vi "Teleop.vi"(10 "Match Info":T1={"Autonomous Elapsed Seconds"=0.0, "TeleOp Elapsed Seconds"=0.0, "Disabled Elapsed Seconds"=0.0, "Visited Autonomous"=FALSE, "Visited TeleOp"=FALSE, "Visited Disabled"=FALSE, "Autonomous Settings"={"Autonomous Style"=enum."Independent", "VI Refnum"=refnum}}, 11 "Call Context":T2) -> ()   [LabVIEW 2019]
doc: "This VI is called for each enabled TeleOp packet received from the DS. It is typically used to read from joysticks and other inputs and update I/O or setpoints for timed control loops. It should complete and return within 20 milliseconds or risk missing DS packets."
uses:
  <vilib>/Rock Robotics/WPI/DriverStation/WPI_DriverStationDerivedRobotMode.ctl
  <vilib>/Rock Robotics/WPI/DriverStation/WPI_DriverStationMatch Info.ctl
  Framework/Robot Global Data.vi
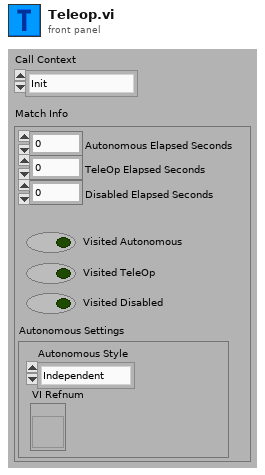
[diagram p1: front panel]
types:
  T1 = typedef "WPI_DriverStationMatch Info.ctl" = cluster{"Autonomous Elapsed Seconds":dbl, "TeleOp Elapsed Seconds":dbl, "Disabled Elapsed Seconds":dbl, "Visited Autonomous":bool, "Visited TeleOp":bool, "Visited Disabled":bool, "Autonomous Settings":cluster{"Autonomous Style":enum16{"Iterative", "Independent"}, "VI Refnum":refnum<vi>}}
  T2 = typedef "WPI_DriverStationDerivedRobotMode.ctl" = enum16{"Init", "Execute", "Stop"}
  T3 = typedef "Command Status Info.ctl" = cluster{"Name":string, "Status":T4, "notifier out":T5}
  T4 = typedef "Completion Status.ctl" = enum16{"Successful", "Aborted", "Incomplete"}
  T5 = typedef "Completion Notifier.ctl" = refnum<notifier>
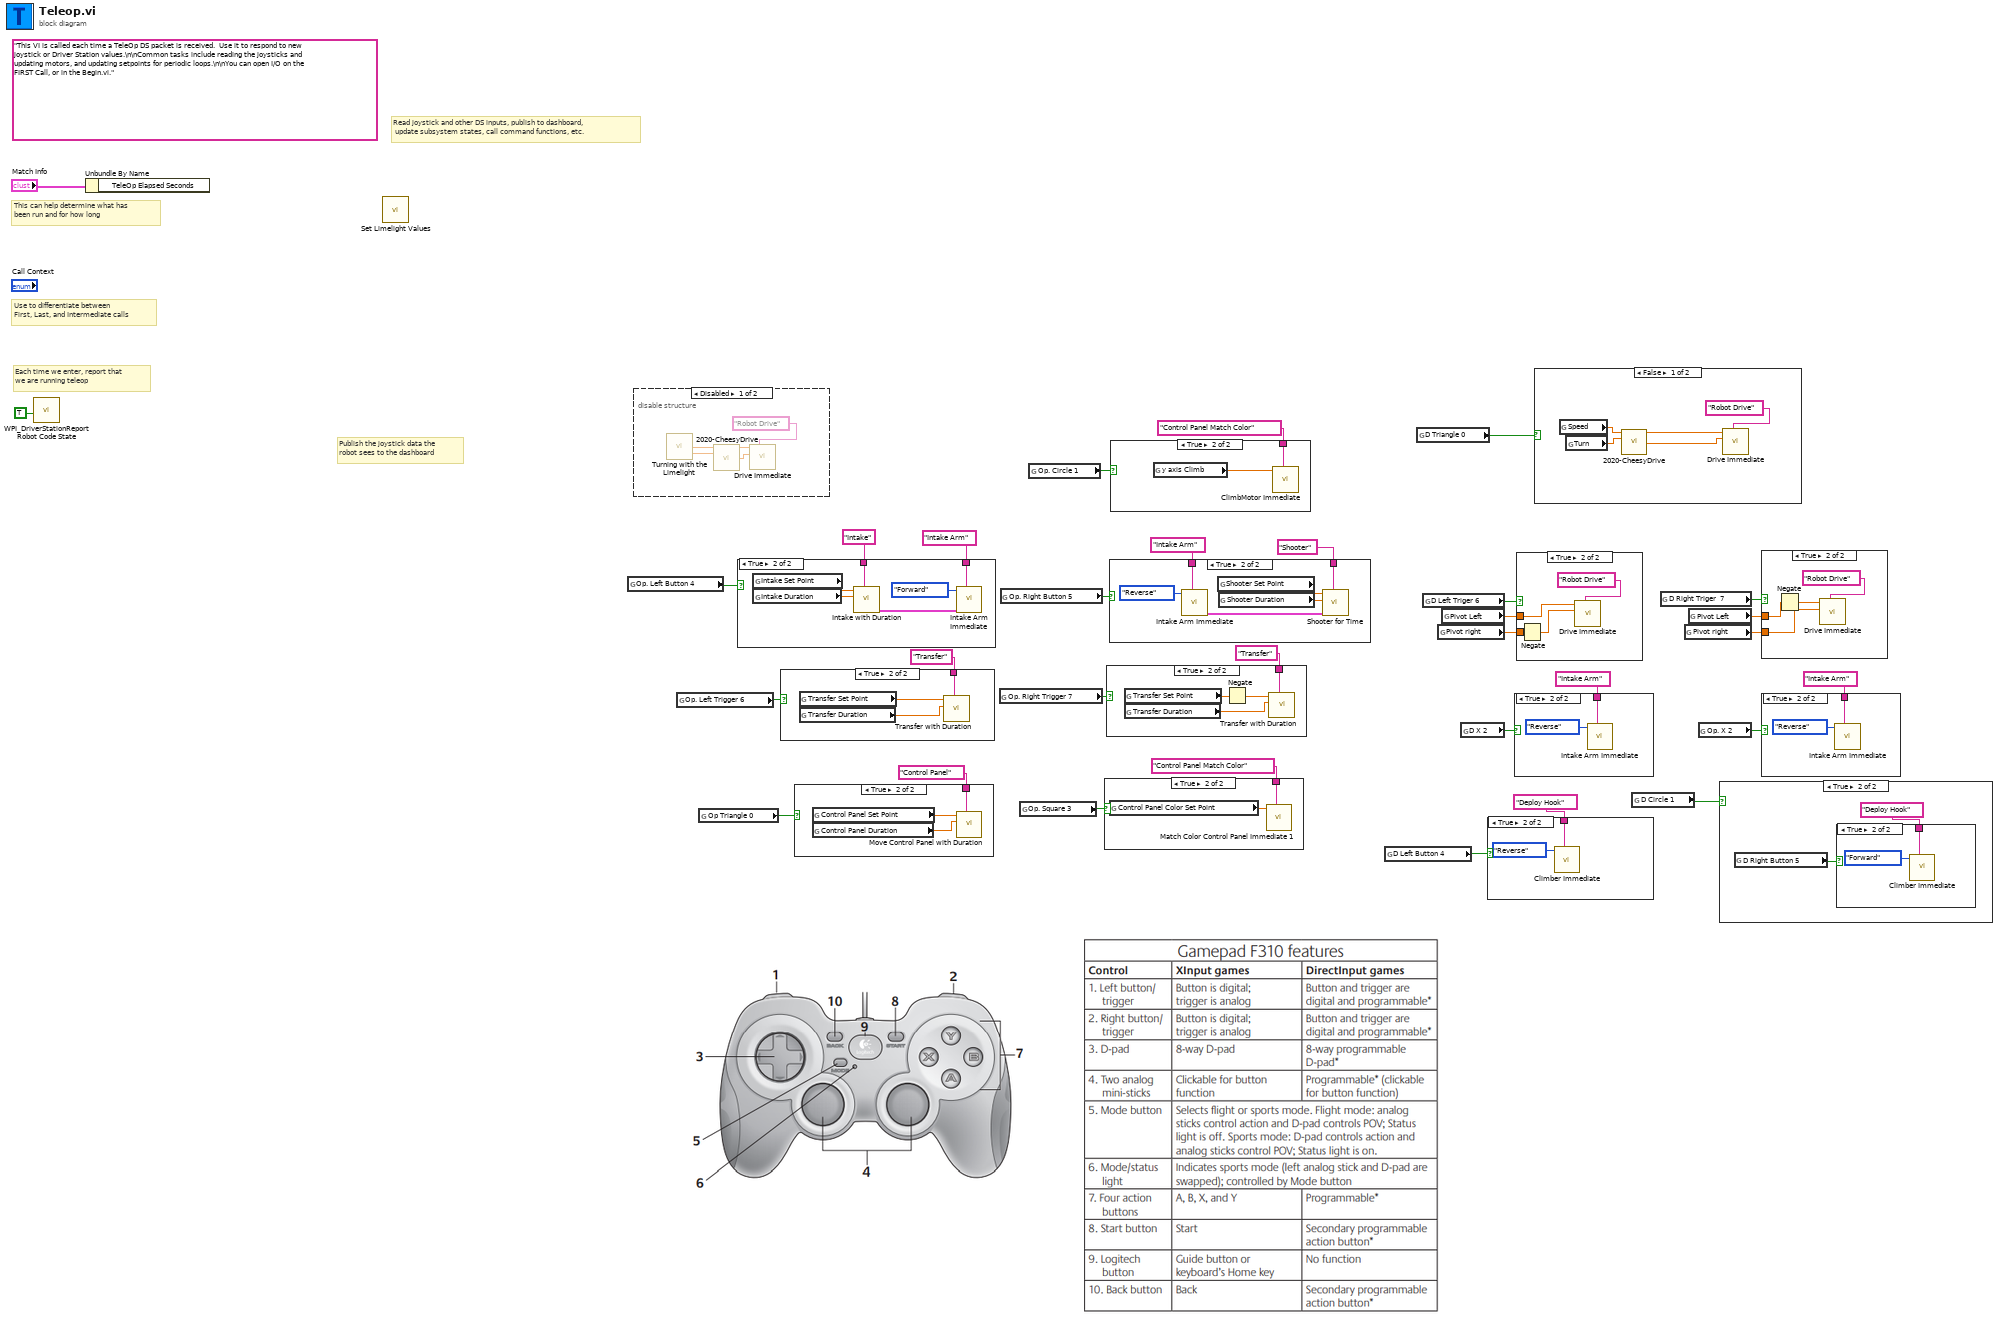
[diagram p0: block diagram]
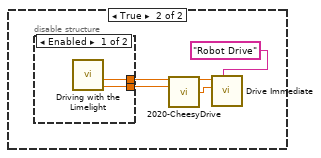
[diagram p8: hidden frame]
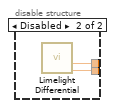
[diagram p9: hidden frame]
diagram:
  (unwired) "This VI is called each time a TeleOp DS packet is received.  Use it to respond to new joystick or Driver Station values.\n\nCommon tasks include reading the joysticks and updating motors, and updating setpoints for periodic loops.\n\nYou can open I/O on the FIRST Call, or in the Begin.vi."
  # "Publish the joystick data the\nrobot sees to the dashboard"
  # "Read joystick and other DS inputs, publish to dashboard,\n update subsystem states, call command functions, etc."
  # "Each time we enter, report that\nwe are running teleop"
  # "Use to differentiate between\nFirst, Last, and Intermediate calls"
  # "This can help determine what has\nbeen run and for how long"
  n1 = call <vilib>:"WPI_DriverStationReport Robot Code State.vi"("TeleOp"=TRUE ("Autonomous")) -> ()  [unwired: 10 in, 1 out]
  n2 = Unbundle By Name("Match Info") -> ()  [unwired: 1 out]
  n3 = call "Set Limelight Values.vi"() -> ()  [unwired: 12 in]
  n4 = global read "Robot Global Data.vi" "Op. Left Button 4"() -> (w30:bool)
  n5 = disable-structure shown="Disabled" {
    frame Disabled {
      n6 = call "Turning with the Limelight.vi"() -> ("TurnCommand"=w36:dbl, "Speed Command"=w37:dbl)  [unwired: 9 in, 1 out]
      n7 = call "2020-CheesyDrive.vi"("Throttle"=w37, "Wheel"=w36) -> ("Left PWM"=w35:dbl, "Right PWM"=w34:dbl)  [unwired: 12 in]
      n8 = call "Drive Immediate.vi"("Description"="Robot Drive", "Right Setpoint"=w34, "Left Setpoint"=w35) -> ()  [unwired: 8 in, 1 out]
    }
    frame Enabled {
    }
  }
  n9 = global read "Robot Global Data.vi" "Op. Left Trigger 6"() -> (w24:bool)
  n10 = global read "Robot Global Data.vi" "Op Triangle 0"() -> (w17:bool)
  n11 = case shown="True" w30 {
    tunnel: "Intake" ("refnum name") -> [_ w43]
    tunnel: "Intake Arm" ("refnum name") -> [_ w39]
    frame False {
    }
    frame True {
      n12 = global read "Robot Global Data.vi" "Intake Set Point"() -> (w42:dbl)
      n13 = global read "Robot Global Data.vi" "Intake Duration"() -> (w41:dbl)
      n14 = call "Intake with Duration.vi"("Description"=w43, "Duration (s)"=w41, "Setpoint"=w42) -> ("Command Info Out"=w38:T3)  [unwired: 8 in]
      n15 = call "Intake Arm Immediate.vi"("Description"=w39, "Command Info In"=w38, "Relay Value"=enum16{"Off", "On", "Forward", "Reverse"}."Forward") -> ()  [unwired: 8 in, 1 out]
    }
  }
  n16 = case shown="True" w24 {
    tunnel: "Transfer" ("refnum name") -> [_ w46]
    frame False {
    }
    frame True {
      n17 = global read "Robot Global Data.vi" "Transfer Set Point"() -> (w45:dbl)
      n18 = global read "Robot Global Data.vi" "Transfer Duration"() -> (w44:dbl)
      n19 = call "Transfer with Duration.vi"("Description"=w46, "Duration (s)"=w44, "Setpoint"=w45) -> ()  [unwired: 8 in, 1 out]
    }
  }
  n20 = case shown="True" w17 {
    tunnel: "Control Panel" ("refnum name") -> [_ w49]
    frame False {
    }
    frame True {
      n21 = global read "Robot Global Data.vi" "Control Panel Set Point"() -> (w48:dbl)
      n22 = global read "Robot Global Data.vi" "Control Panel Duration"() -> (w47:dbl)
      n23 = call "Move Control Panel with Duration.vi"("Description"=w49, "Duration (s)"=w47, "Setpoint"=w48) -> ()  [unwired: 8 in, 1 out]
    }
  }
  n24 = global read "Robot Global Data.vi" "Op. Right Trigger 7"() -> (w25:bool)
  n25 = global read "Robot Global Data.vi" "Op. Right Button 5"() -> (w26:bool)
  n26 = global read "Robot Global Data.vi" "Op. Square 3"() -> (w14:bool)
  n27 = global read "Robot Global Data.vi" "Op. Circle 1"() -> (w2:bool)
  n28 = case shown="True" w14 {
    tunnel: "Control Panel Match Color" ("refnum name") -> [_ w51]
    frame False {
    }
    frame True {
      n29 = global read "Robot Global Data.vi" "Control Panel Color Set Point"() -> (w50:dbl)
      n30 = call "Match Color Control Panel Immediate 1.vi"("Description"=w51, "Setpoint"=w50) -> ()  [unwired: 9 in, 1 out]
    }
  }
  n31 = case shown="True" w25 {
    tunnel: "Transfer" ("refnum name") -> [_ w55]
    frame False {
    }
    frame True {
      n32 = global read "Robot Global Data.vi" "Transfer Set Point"() -> (w53:dbl)
      n33 = global read "Robot Global Data.vi" "Transfer Duration"() -> (w52:dbl)
      n34 = Negate(x=w53) -> (-x=w54:dbl)
      n35 = call "Transfer with Duration.vi"("Description"=w55, "Duration (s)"=w52, "Setpoint"=w54) -> ()  [unwired: 8 in, 1 out]
    }
  }
  n36 = case shown="True" w26 {
    tunnel: "Shooter" ("refnum name") -> [_ w61]
    tunnel: "Intake Arm" ("refnum name") -> [_ w56]
    frame False {
    }
    frame True {
      n37 = call "Intake Arm Immediate.vi"("Description"=w56, "Relay Value"=enum16{"Off", "On", "Forward", "Reverse"}."Reverse") -> ("Command Info Out"=w57:T3)  [unwired: 9 in]
      n38 = global read "Robot Global Data.vi" "Shooter Set Point"() -> (w60:dbl)
      n39 = global read "Robot Global Data.vi" "Shooter Duration"() -> (w59:dbl)
      n40 = call "Shooter for Time.vi"("Description"=w61, "Command Info In"=w57, "Duration (s)"=w59, "Setpoint"=w60) -> ()  [unwired: 7 in, 1 out]
    }
  }
  n41 = case shown="True" w2 {
    tunnel: "Control Panel Match Color" ("refnum name") -> [_ w63]
    frame False {
    }
    frame True {
      n42 = global read "Robot Global Data.vi" "y axis Climb"() -> (w62:dbl)
      n43 = call "ClimbMotor Immediate.vi"("Description"=w63, "Setpoint"=w62) -> ()  [unwired: 9 in, 1 out]
    }
  }
  n44 = global read "Robot Global Data.vi" "D Left Button 4"() -> (w7:bool)
  n45 = global read "Robot Global Data.vi" "D Triangle 0"() -> (w8:bool)
  n46 = global read "Robot Global Data.vi" "D Left Triger 6"() -> (w22:bool)
  n47 = global read "Robot Global Data.vi" "Pivot right"() -> (w11:dbl)
  n48 = global read "Robot Global Data.vi" "Pivot Left"() -> (w12:dbl)
  n49 = global read "Robot Global Data.vi" "D X 2"() -> (w15:bool)
  n50 = case shown="True" w7 {
    tunnel: "Deploy Hook" ("refnum name") -> [_ w64]
    frame False {
    }
    frame True {
      n51 = call "Climber Immediate.vi"("Description"=w64, "Value"=enum16{"Off", "On", "Forward", "Reverse"}."Reverse" ("Relay Value")) -> ()  [unwired: 9 in, 1 out]
    }
  }
  n52 = case shown="True" w15 {
    tunnel: "Intake Arm" ("refnum name") -> [_ w66]
    frame False {
    }
    frame True {
      n53 = call "Intake Arm Immediate.vi"("Description"=w66, "Relay Value"=enum16{"Off", "On", "Forward", "Reverse"}."Reverse") -> ()  [unwired: 9 in, 1 out]
    }
  }
  n54 = case shown="True" w22 {
    tunnel: w12 -> [_ w70]
    tunnel: w11 -> [_ w69]
    frame False {
    }
    frame True {
      n55 = Negate(x=w69) -> (-x=w68:dbl)
      n56 = call "Drive Immediate.vi"("Description"="Robot Drive", "Right Setpoint"=w68, "Left Setpoint"=w70) -> ()  [unwired: 8 in, 1 out]
    }
  }
  n57 = case shown="False" w8 {
    frame False {
      n58 = global read "Robot Global Data.vi" "Speed"() -> (w73:dbl)
      n59 = global read "Robot Global Data.vi" "Turn"() -> (w74:dbl)
      n60 = call "2020-CheesyDrive.vi"("Throttle"=w73, "Wheel"=w74) -> ("Left PWM"=w75:dbl, "Right PWM"=w76:dbl)  [unwired: 12 in]
      n61 = call "Drive Immediate.vi"("Description"="Robot Drive", "Right Setpoint"=w76, "Left Setpoint"=w75) -> ()  [unwired: 8 in, 1 out]
    }
    frame True {
      n62 = disable-structure shown="Enabled" {
        disable-tunnel: [w83 w84] -> w77
        disable-tunnel: [w82 w85] -> w78
        frame Enabled {
          n63 = call "Driving with the Limelight.vi"() -> ("TurnCommand"=w83:dbl, "SpeedCommand"=w82:dbl)  [unwired: 9 in, 1 out]
        }
        frame Disabled {
          n64 = call "Limelight Differential.vi"() -> ("DriveCommand"=w84:dbl, "SteerCommand"=w85:dbl)  [unwired: 9 in, 1 out]
        }
      }
      n65 = call "2020-CheesyDrive.vi"("Throttle"=w78, "Wheel"=w77) -> ("Left PWM"=w80:dbl, "Right PWM"=w81:dbl)  [unwired: 12 in]
      n66 = call "Drive Immediate.vi"("Description"="Robot Drive", "Right Setpoint"=w81, "Left Setpoint"=w80) -> ()  [unwired: 8 in, 1 out]
    }
  }
  n67 = global read "Robot Global Data.vi" "D Circle 1"() -> (w1:bool)
  n68 = global read "Robot Global Data.vi" "D Right Triger  7"() -> (w21:bool)
  n69 = global read "Robot Global Data.vi" "Pivot right"() -> (w9:dbl)
  n70 = global read "Robot Global Data.vi" "Pivot Left"() -> (w10:dbl)
  n71 = global read "Robot Global Data.vi" "Op. X 2"() -> (w5:bool)
  n72 = case shown="True" w1 {
    frame False {
    }
    frame True {
      n73 = global read "Robot Global Data.vi" "D Right Button 5"() -> (w86:bool)
      n74 = case shown="True" w86 {
        tunnel: "Deploy Hook" ("refnum name") -> [_ w88]
        frame False {
        }
        frame True {
          n75 = call "Climber Immediate.vi"("Description"=w88, "Value"=enum16{"Off", "On", "Forward", "Reverse"}."Forward" ("Relay Value")) -> ()  [unwired: 9 in, 1 out]
        }
      }
    }
  }
  n76 = case shown="True" w21 {
    tunnel: w10 -> [_ w92]
    tunnel: w9 -> [_ w91]
    frame False {
    }
    frame True {
      n77 = Negate(x=w92) -> (-x=w90:dbl)
      n78 = call "Drive Immediate.vi"("Description"="Robot Drive", "Right Setpoint"=w91, "Left Setpoint"=w90) -> ()  [unwired: 8 in, 1 out]
    }
  }
  n79 = case shown="True" w5 {
    tunnel: "Intake Arm" ("refnum name") -> [_ w94]
    frame False {
    }
    frame True {
      n80 = call "Intake Arm Immediate.vi"("Description"=w94, "Relay Value"=enum16{"Off", "On", "Forward", "Reverse"}."Reverse") -> ()  [unwired: 9 in, 1 out]
    }
  }
